vi "set filter (section).vi"(5 "Use AND Logic? (False)":bool, 7 "Combine Existing (False)":bool, 8 "error in (no error)":errorcluster, 10 "Type":enum16{"All", "Target", "Model"}(ring), 11 "alias-tree in":refnum<class "alias-tree.lvclass">) -> (0 "error out":errorcluster, 3 "alias-tree out":refnum<class "alias-tree.lvclass">)   [LabVIEW 2017, in "vs-tree-utility.lvlib" / "alias-tree.lvclass"]
uses:
  alias-tree.lvclass
  NationalInstruments.VeriStand.SystemStorage
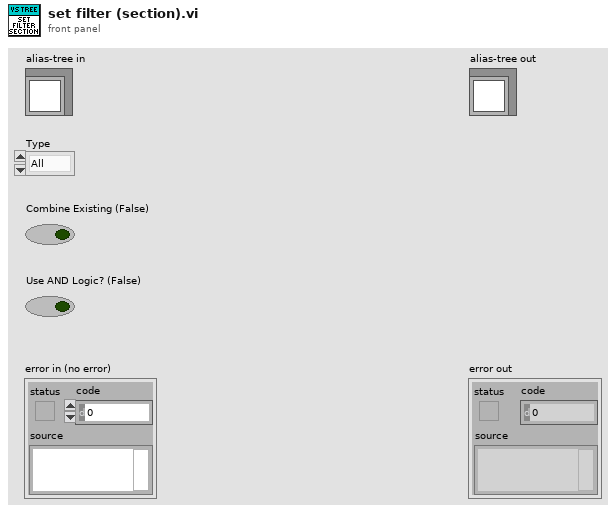
[diagram p1: front panel]
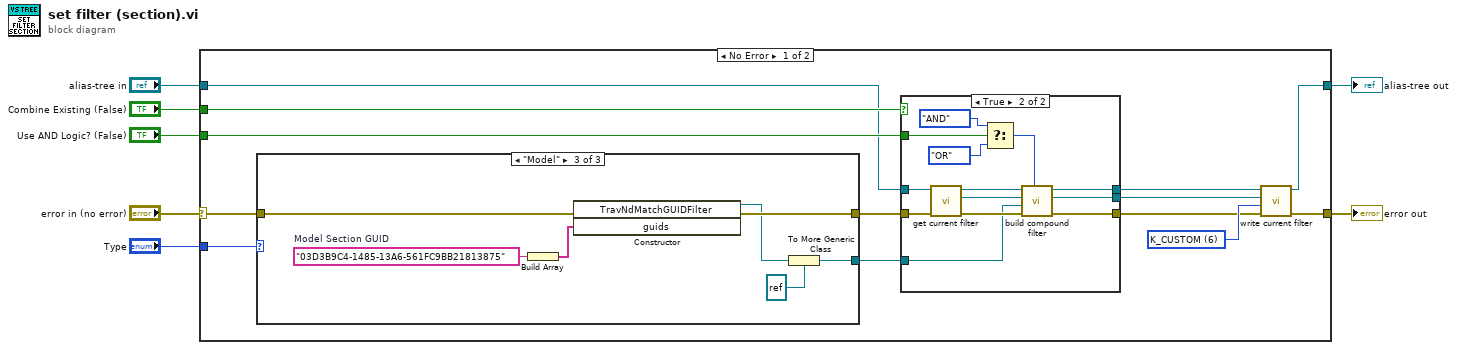
[diagram p0: block diagram]
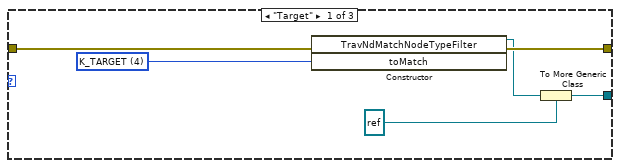
[diagram p3: hidden frame]
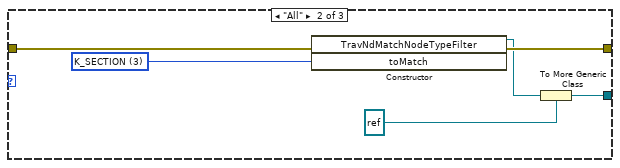
[diagram p4: hidden frame]
diagram:
  n1 = case shown="No Error" "error in (no error)" {
    selector: "error in (no error)" -> [w20 w57]
    tunnel: [w16 w57] -> w6
    tunnel: [w18 w56] -> w4
    tunnel: "alias-tree in" -> [w8 w56]
    tunnel: "Type" -> [w19 _]
    tunnel: "Combine Existing (False)" -> [w15 _]
    tunnel: "Use AND Logic? (False)" -> [w14 _]
    frame No Error {
      w17 = u8 6 items=["K_CHAN_R", "K_CHAN_W", "K_CHAN_RW", "K_CHAN_VOLT", "K_CHAN_FAULT", "K_ALL", "K_CUSTOM", "K_CHAN_R_VIS", "K_CHAN_W_VIS", "K_CHAN_RW_VIS", "K_CHAN_VOLT_VIS", "K_CHAN_FAULT_VIS", "K_WAVE", "K_WAVE_VIS", "K_WAVE_DBL", "K_WAVE_CDB", "K_WAVE_DBL_VIS", "K_WAVE_CDB_VIS"] ("filterType")
      n2 = case shown="\"Model\"" w19 {
        tunnel: w20 -> [w42 w48 w55]
        tunnel: [w41 w47 w54] -> w13
        tunnel: [w38 w44 w51] -> w10
        frame "Target" {
          w37 = 4 items=["K_BASE", "K_ALIAS", "K_CHANNEL", "K_SECTION", "K_TARGET", "K_TARGETSECTION", "K_ROOT", "K_WAVEFORM", "K_PARAMETER"] ("toMatch")
          n3 = constructor class="TravNdMatchNodeTypeFilter"(error in=w42, "toMatch"=w37) -> (reference out=w40:refnum<k24>, error out=w41:errorcluster)  [unwired: 2 in, 2 out]
          n4 = To More Generic Class(target class=refnum<k24> refnum ("customFilter"), reference=w40) -> (generic class reference=w38:refnum<k24>)
        }
        frame "All" {
          w43 = 3 items=["K_BASE", "K_ALIAS", "K_CHANNEL", "K_SECTION", "K_TARGET", "K_TARGETSECTION", "K_ROOT", "K_WAVEFORM", "K_PARAMETER"] ("toMatch")
          n5 = constructor class="TravNdMatchNodeTypeFilter"(error in=w48, "toMatch"=w43) -> (reference out=w46:refnum<k24>, error out=w47:errorcluster)  [unwired: 2 in, 2 out]
          n6 = To More Generic Class(target class=refnum<k24> refnum ("customFilter"), reference=w46) -> (generic class reference=w44:refnum<k24>)
        }
        frame "Model" {
          w50 = "03D3B9C4-1485-13A6-561FC9BB21813875"  # Model Section GUID
          n7 = Build Array(w50) -> (w49:string[])
          n8 = constructor class="TravNdMatchGUIDFilter"(error in=w55, "guids"=w49) -> (reference out=w53:refnum<k24>, error out=w54:errorcluster)  [unwired: 2 in, 2 out]
          n9 = To More Generic Class(target class=refnum<k24> refnum ("customFilter"), reference=w53) -> (generic class reference=w51:refnum<k24>)
        }
      }
      n10 = case shown="True" w15 {
        tunnel: w14 -> [_ w31]
        tunnel: w13 -> [w23 w36]
        tunnel: [w23 w34] -> w12
        tunnel: [w22 w25] -> w11
        tunnel: w10 -> [w22 w32]
        tunnel: [w21 w26] -> w9
        tunnel: w8 -> [w21 w24]
        frame False {
        }
        frame True {
          n11 = call "get current filter.vi"("error in (no error)"=w36, "alias-tree in"=w24) -> ("error out"=w35:errorcluster, "display filter"=w33:refnum<k24>, "alias-tree out"=w27:refnum<class "alias-tree.lvclass">)  [unwired: 7 in]
          n12 = Select(t=enum16{"AND", "OR"}."AND" ("Type (OR)"), s=w31, f=enum16{"AND", "OR"}."OR" ("Type (OR)")) -> (s? t:f=w28:enum16{"AND", "OR"})
          n13 = call-dynamic "build compound filter.vi"("Type (OR)"=w28, "error in (no error)"=w35, "Filter B"=w32, "Filter A"=w33, "alias-tree in"=w27) -> ("error out"=w34:errorcluster, "Compound Filter"=w25:refnum<k24>, "alias-tree out"=w26:refnum<class "alias-tree.lvclass">)  [unwired: 4 in]
        }
      }
      n14 = call-dynamic "write current filter.vi"("error in (no error)"=w12, "filterType"=w17, "Filter"=w11, "alias-tree in"=w9) -> ("error out"=w16:errorcluster, "alias-tree out"=w18:refnum<class "alias-tree.lvclass">)  [unwired: 6 in]
    }
    frame Error {
    }
  }
  "error out" <- w6
  "alias-tree out" <- w4
